vi "Encoder Control Logic.vi"(8 "Prev Phase B (State Bit 1)":bool, 9 "Prev Phase A (State Bit 0)":bool, 10 "Phase B":bool, 11 "Phase A":bool) -> (1 "Count?":bool, 2 "Backward?":bool, 3 "Error Occurred?":bool)   [LabVIEW 2013]
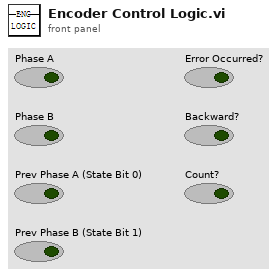
[diagram p1: front panel]
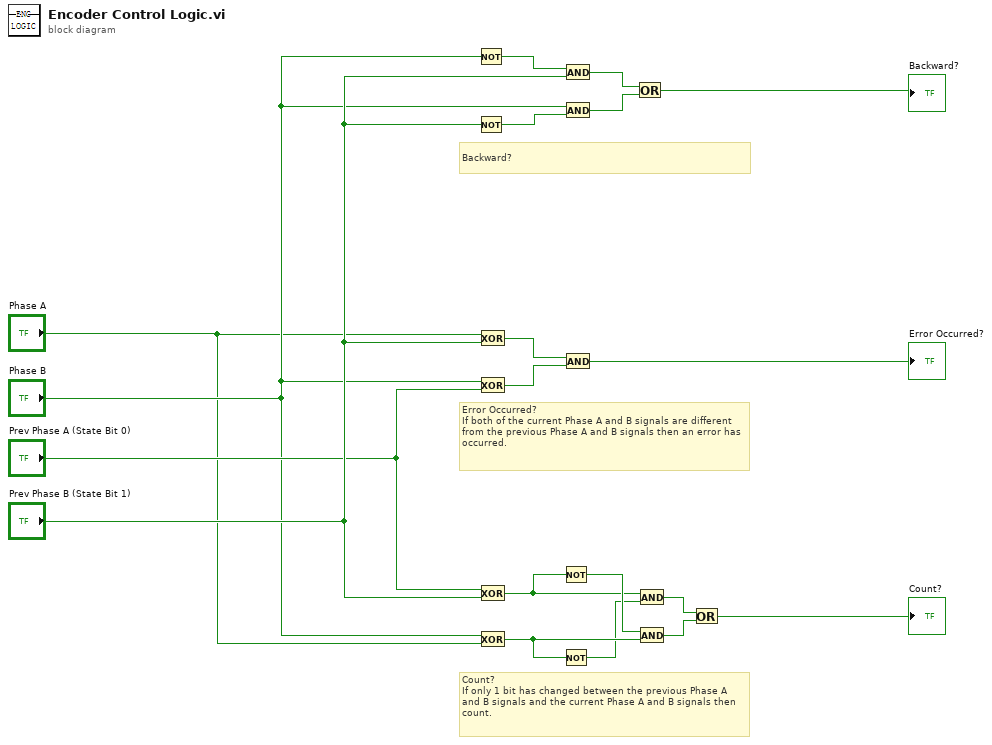
[diagram p0: block diagram]
diagram:
  # "Backward?"
  # "Count?\nIf only 1 bit has changed between the previous Phase A and B signals and the current Phase A and B signals then count."
  # "Error Occurred?\nIf both of the current Phase A and B signals are different from the previous Phase A and B signals then an error has occurred."
  n1 = Not(x="Phase B") -> (.not. x?=w16:bool)
  n2 = Not(x="Prev Phase B (State Bit 1)") -> (.not. x?=w15:bool)
  n3 = Exclusive Or(1:"Prev Phase B (State Bit 1)", 2:"Phase A") -> (0:w4:bool)
  n4 = Exclusive Or(1:"Prev Phase A (State Bit 0)", 2:"Phase B") -> (0:w5:bool)
  n5 = Exclusive Or(1:"Prev Phase B (State Bit 1)", 2:"Prev Phase A (State Bit 0)") -> (0:w6:bool)
  n6 = Exclusive Or(1:"Phase A", 2:"Phase B") -> (0:w8:bool)
  n7 = Not(x=w6) -> (.not. x?=w9:bool)
  n8 = Not(x=w8) -> (.not. x?=w7:bool)
  n9 = And(x=w16, y="Prev Phase B (State Bit 1)") -> (x .and. y?=w13:bool)
  n10 = And(x="Phase B", y=w15) -> (x .and. y?=w14:bool)
  n11 = And(x=w4, y=w5) -> (x .and. y?=→"Error Occurred?":bool)
  n12 = Or(x=w13, y=w14) -> (x .or. y?=→"Backward?":bool)
  n13 = And(x=w6, y=w7) -> (x .and. y?=w10:bool)
  n14 = And(x=w9, y=w8) -> (x .and. y?=w11:bool)
  n15 = Or(x=w10, y=w11) -> (x .or. y?=→"Count?":bool)
